vi "Actor Core.vi"(8 "error in":errorcluster, 11 "Description Panel in":refnum<class "Description Panel.lvclass">) -> (0 "error out":errorcluster, 3 "Actor out":refnum<class "Actor.lvclass">)   [LabVIEW 2017, in "2. Basic Panel Actors.lvlib" / "Description Panel.lvclass"]
doc: "The user interface for this panel.\n----\nCopyright: MGI 2016\nAuthor: Derek Trepanier"
uses:
  Description Panel.lvclass
  panel-manager/Source/MGI-Panel Manager.lvlib
  <vilib>/ActorFramework/Stop Msg/Stop Msg.lvclass
  panel-manager/Source/Panel/Subpanel/Subpanel.vi
  panel-manager/Source/Panel/Subpanel/Subpanel.lvclass
  panel-actors/Source/Panel Actor/Panel Actor.lvclass
  panel-manager/Source/Panel/Panel.lvclass
  D:/software/LabView_PanelManager/panel-manager/Source/Panel/Panel.lvclass
  panel-manager/Source/Init Waiter/Init Waiter.lvclass
  D:/software/LabView_PanelManager/panel-actors/Source/Panel Actor/Panel Actor.lvclass
  C:/Program Files (x86)/National Instruments/LabVIEW 2017/vi.lib/ActorFramework/Actor/Actor.lvclass
  <vilib>/ActorFramework/Actor/Actor.lvclass
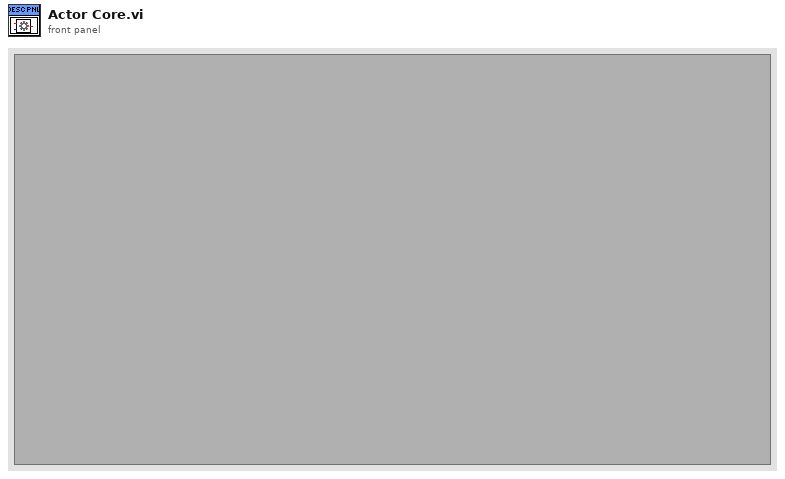
[diagram p1: front panel]
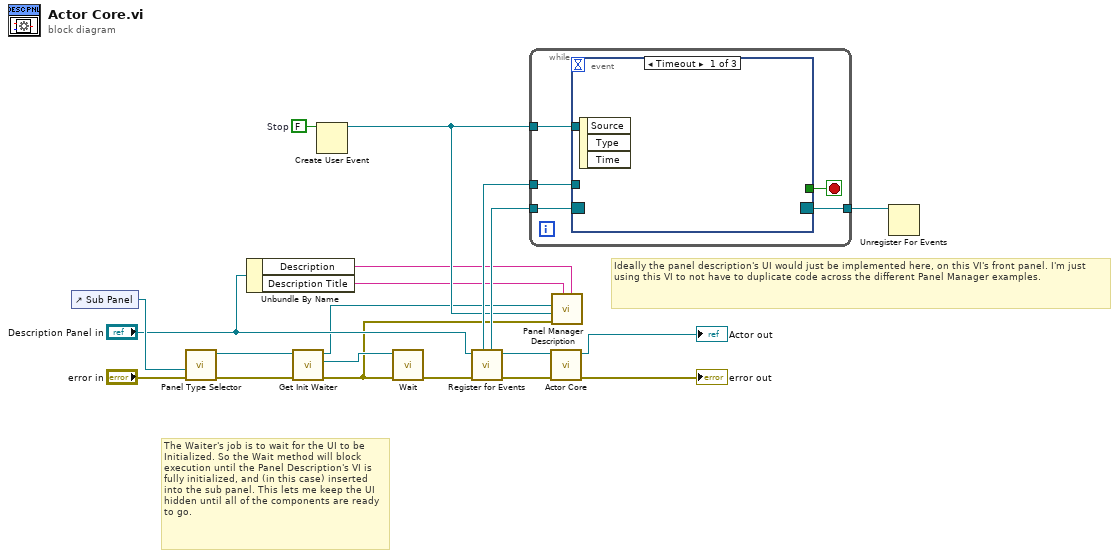
[diagram p0: block diagram]
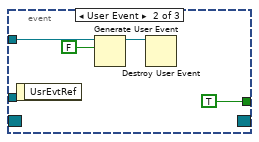
[diagram p2: hidden frame]
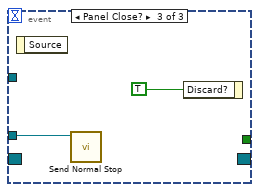
[diagram p3: hidden frame]
diagram:
  w19 = FALSE  # Stop
  # "The Waiter's job is to wait for the UI to be Initialized. So the Wait method will block execution until the Panel Description's VI is fully initialized, and (in this case) inserted into the sub panel. This lets me keep the UI hidden until all of the components are ready to go."
  # "Ideally the panel description's UI would just be implemented here, on this VI's front panel. I'm just using this VI to not have to duplicate code across the different Panel Manager examples."
  n1 = control-ref of="Sub Panel"() -> (w12:refnum<vi>)
  n2 = call-poly "Panel Type Selector.vi"("Error In"="error in", "Sub Panel"=w12) -> ("Error Out"=w18:errorcluster, "Subpanel Out"=w17:refnum<class "Subpanel.lvclass">)  [unwired: 8 in]
  n3 = Unbundle By Name("Description Panel in") -> ("Description"=w1:string, "Description Title"=w2:string)
  n4 = call "Get Init Waiter.vi"("Error In"=w18, "Panel In"=w17) -> ("Error Out"=w5:errorcluster, "Init Waiter"=w14:refnum<class "Init Waiter.lvclass">, "Panel Out"=w3:refnum<class "Subpanel.lvclass">)  [unwired: 7 in]
  n5 = Create User Event(user event datatype=w19) -> (user event=w4:refnum<user-event>)  [unwired: 1 in, 1 out]
  n6 = call "Wait.vi"("Error In"=w5, "Init Waiter in"=w14) -> ("Error Out"=w15:errorcluster)  [unwired: 7 in, 2 out]
  n7 = call "Register for Events.vi"("Error In"=w15, "Panel Actor in"="Description Panel in") -> ("Error Out"=w11:errorcluster, "Panel Actor out"=w10:refnum<class "Description Panel.lvclass">, "Pnl Actor"=w8:refnum<event-registration>, "Self Enqueuer"=w7:refnum<class "Message Enqueuer.lvclass">)  [unwired: 5 in, 1 out]
  n8 = while {
    tunnel: w8 -> [w25]
    tunnel: [w23] -> w6
    tunnel: w4 -> [w22]
    tunnel: w7 -> [w21]
    stop <- w24 stop-if-true
    n9 = event shown="[0] Timeout" {
      selector: w25 -> [_ _ _]
      dyn-events: [_ _ _] -> w23
      timeout: _ -> [_ _ _]
      tunnel: [_ TRUE _] -> w24
      tunnel: w22 -> [_ w26 _]
      tunnel: w21 -> [_ _ w30]
      event Timeout {
        n10 = event-data() -> ()  [unwired: 1 in, 3 out]
      }
      event User Event {
        n11 = event-data() -> ()  [unwired: 1 in, 1 out]
        n12 = Generate User Event(user event=w26, event data cluster=FALSE ("event data")) -> (user event out=w28:refnum<user-event>)  [unwired: 2 in, 1 out]
        n13 = Destroy User Event(user event=w28) -> ()  [unwired: 1 in, 1 out]
      }
      event Panel Close? {
        n14 = event-data() -> ()  [unwired: 1 in, 1 out]
        n15 = call <vilib>:"Send Normal Stop.vi"("Message Enqueuer"=w30) -> ()  [unwired: 10 in, 1 out]
        n16 = event-data("Discard?"=TRUE) -> ()  [unwired: 1 in, 1 out]
      }
    }
  }
  n17 = call-parent "Actor Core.vi"("error in"=w11, "Panel Actor in"=w10) -> ("error out"=→"error out":errorcluster, "Actor out"=→"Actor out":refnum<class "Actor.lvclass">)  [unwired: 8 in]
  n18 = call "Panel Manager Description.vi"("Description"=w1, "Description Title"=w2, "error in (no error)"=w5, "Stop Event"=w4, "Panel"=w3) -> ()  [unwired: 6 in, 1 out]
  n19 = Unregister For Events(event registration refnum=w6) -> ()  [unwired: 1 in, 1 out]
